vi "Analog Gen Cfg Popup.vi"(8 "error in (no error)":errorcluster, 11 "config file in":path caption="Configuration File") -> (0 "error out":errorcluster, 3 "config file out":path caption="Configuration File")   [LabVIEW 2021, in "Audio Popup UI.lvlib"]
uses:
  Audio Popup UI.lvlib
  service/generation/controls/analog output settings.ctl
  service/generation/controls/terminal configuration.ctl
  <vilib>/Utility/miscctls.llb/LVPointTypeDef.ctl
  analog gen settings/Analog Gen Settings.lvlib
  service/generation/controls/AudioGenTypeDefs.lvlib
panel:
  in  "terminal configuration":T1 caption="Terminal configuration"
  in  "range":dbl=2.0 caption="Output range"
  out "output settings":T2={"output rate"=0.0, "range"=0.0, "terminal configuration"=enum."Pseudodifferential", "output impedance"=0.0, "common mode offset"=0.0, "pure tone mode"=FALSE}
  in  "Save":bool
  in  "output rate":dbl=2.0 caption="Output rate"
  # "Analog Output Configuration"
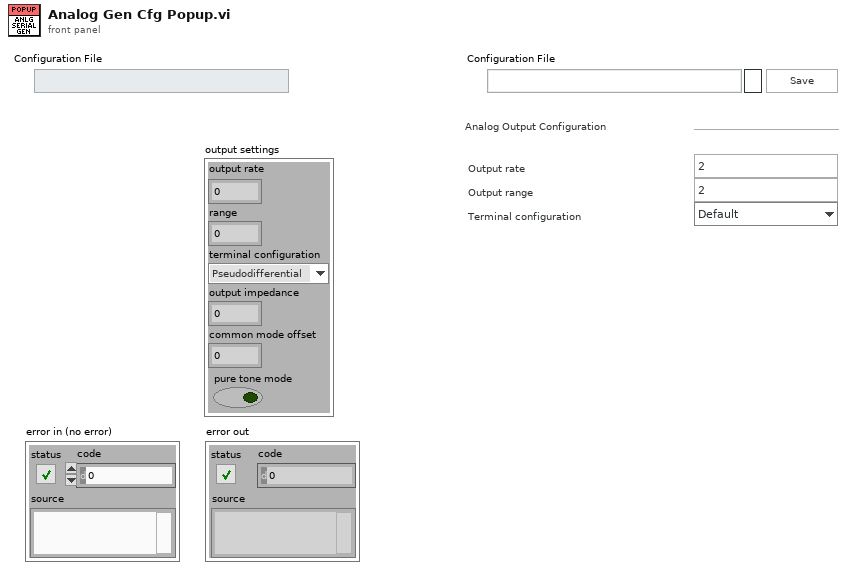
[diagram p1: front panel]
types:
  T1 = typedef "AudioGenTypeDefs.lvlib/terminal configuration.ctl" = enum32{"Default", "RSE", "Differential", "Pseudodifferential"}
  T2 = typedef "AudioGenTypeDefs.lvlib/analog output settings.ctl" = cluster{"output rate":dbl, "range":dbl, "terminal configuration":T1, "output impedance":dbl, "common mode offset":dbl, "pure tone mode":bool}
  T3 = typedef "LVPointTypeDef.ctl" = cluster{"Horizontal":i16, "Vertical":i16}
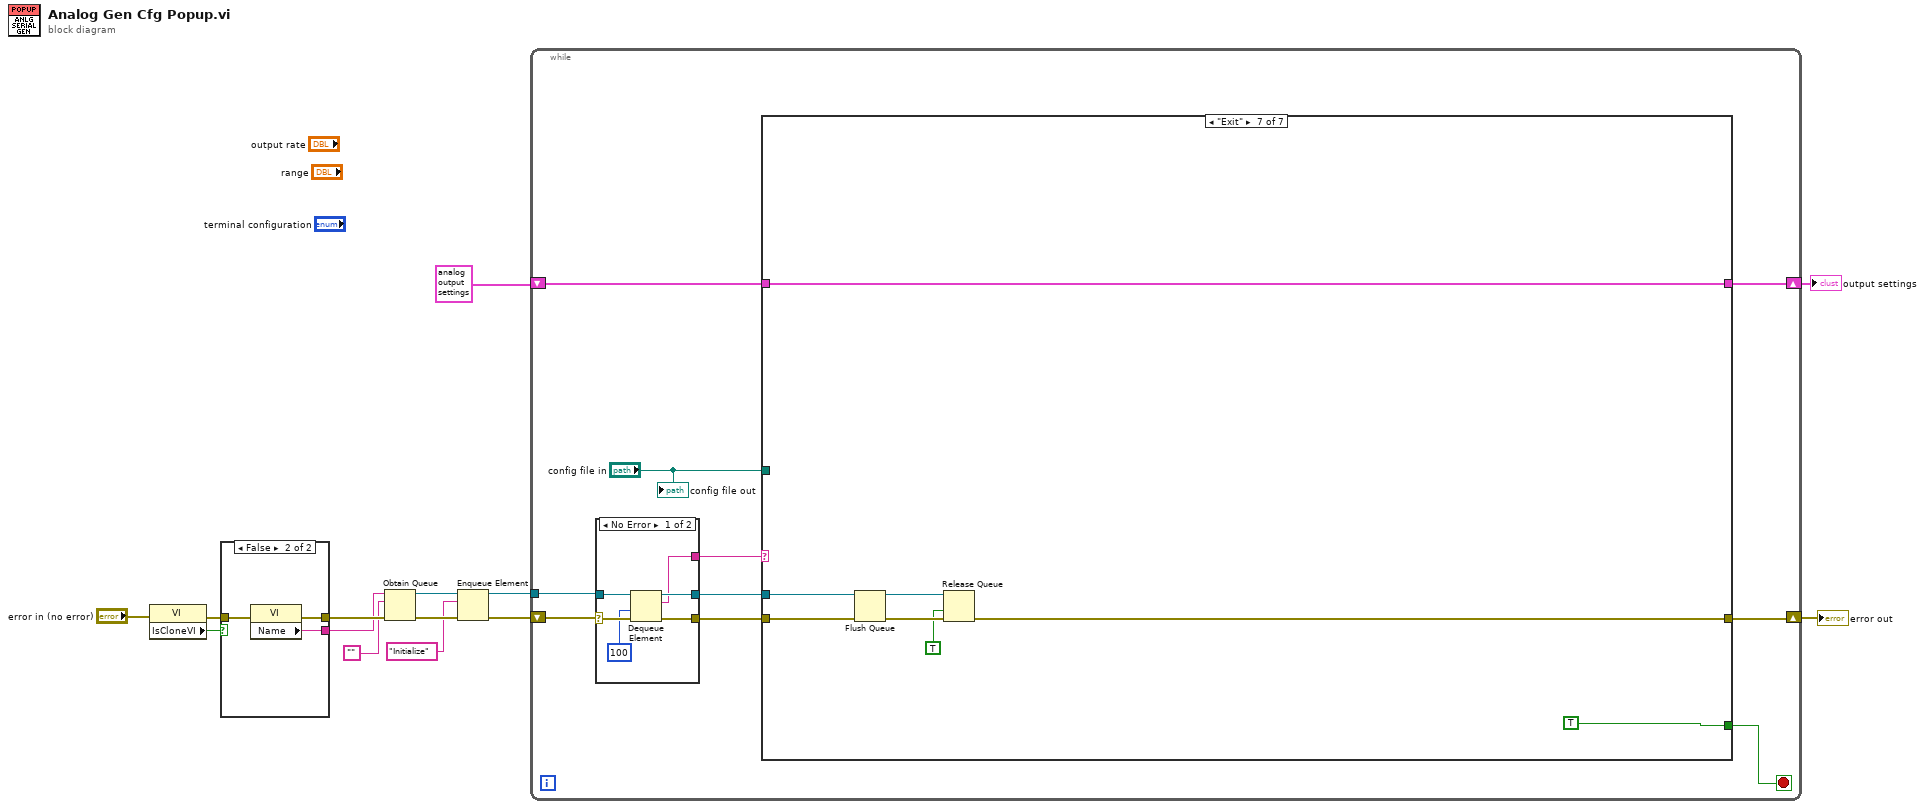
[diagram p0: block diagram]
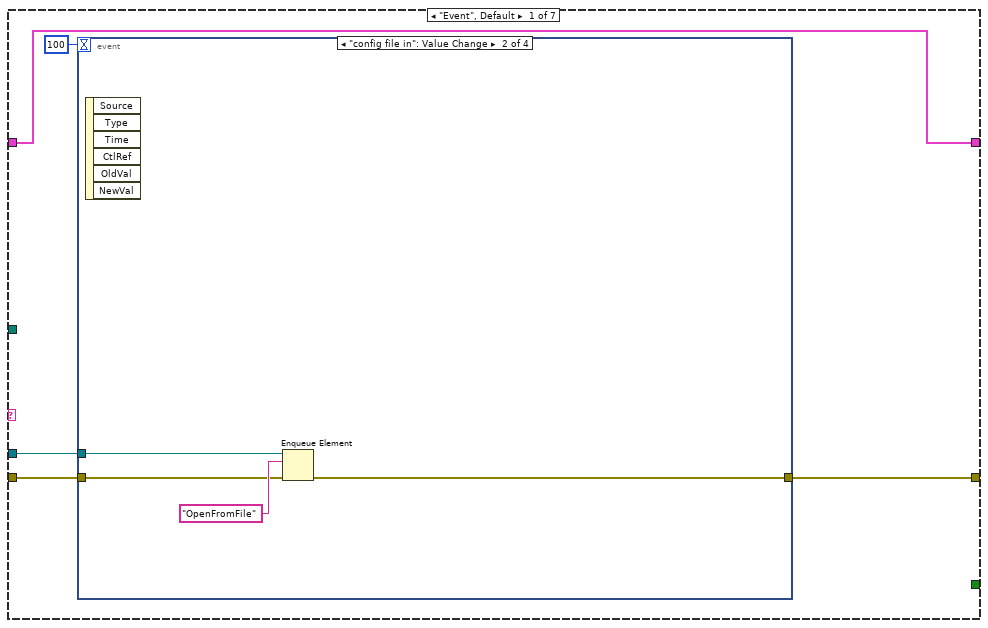
[diagram p2: hidden frame]
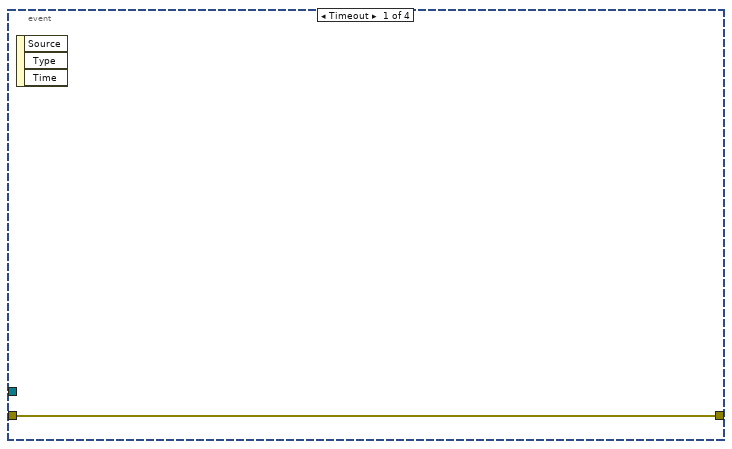
[diagram p3: hidden frame]
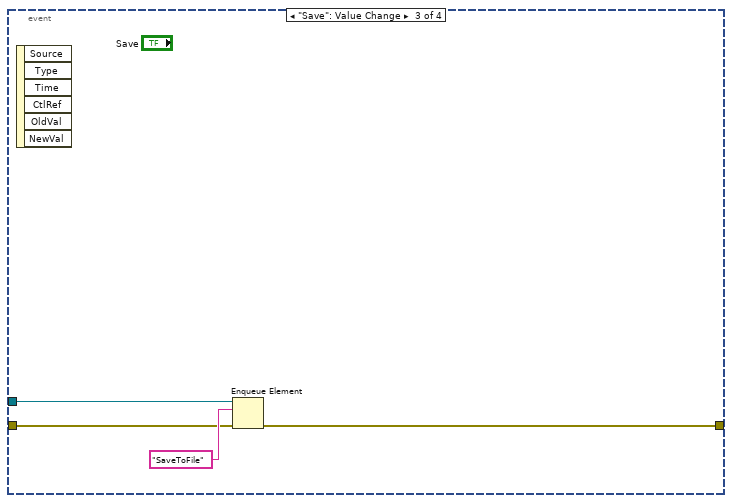
[diagram p4: hidden frame]
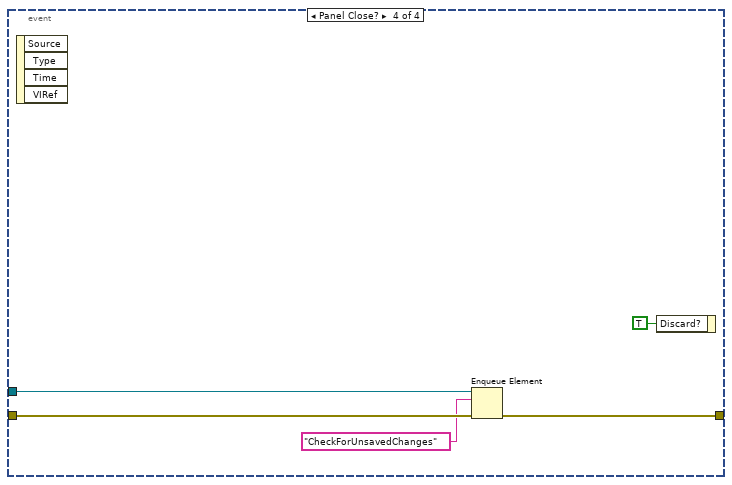
[diagram p5: hidden frame]
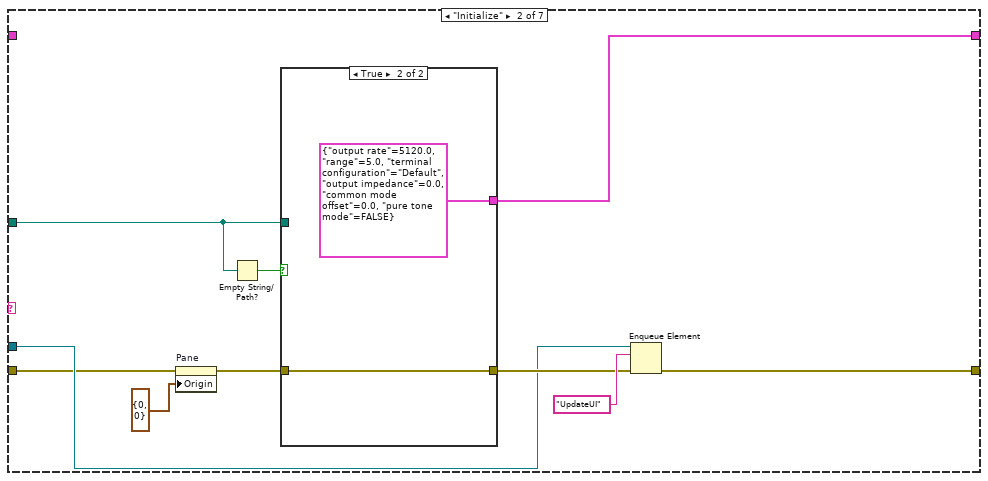
[diagram p6: hidden frame]
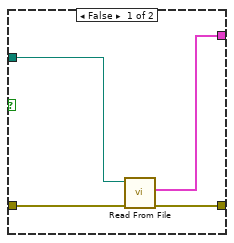
[diagram p7: hidden frame]
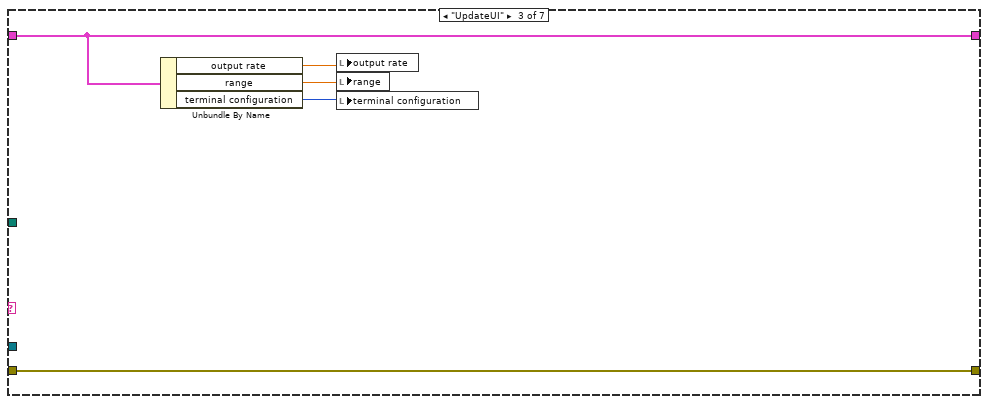
[diagram p8: hidden frame]
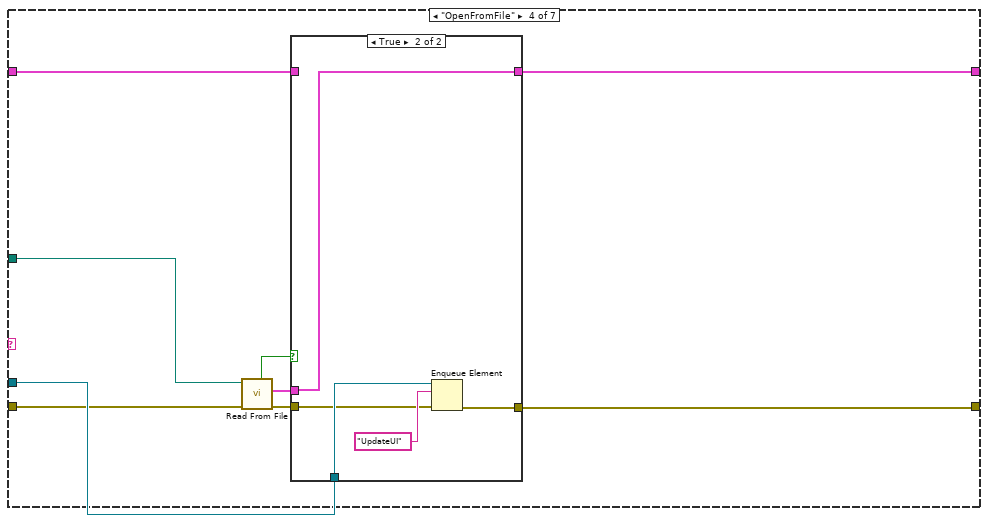
[diagram p9: hidden frame]
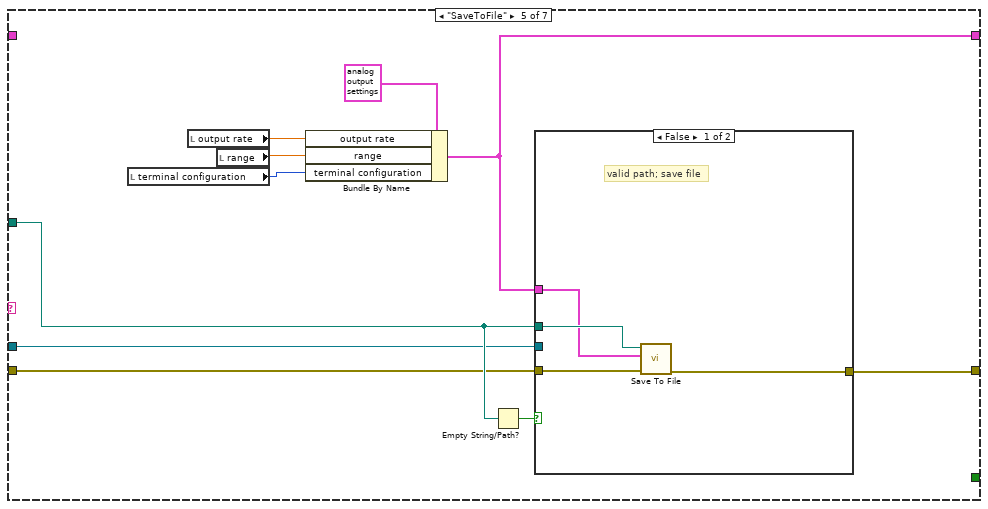
[diagram p11: hidden frame]
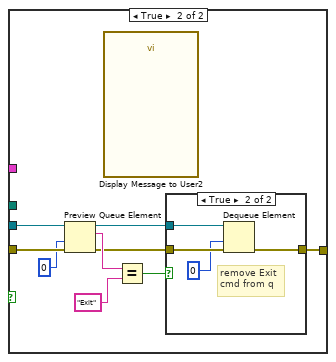
[diagram p12: hidden frame]
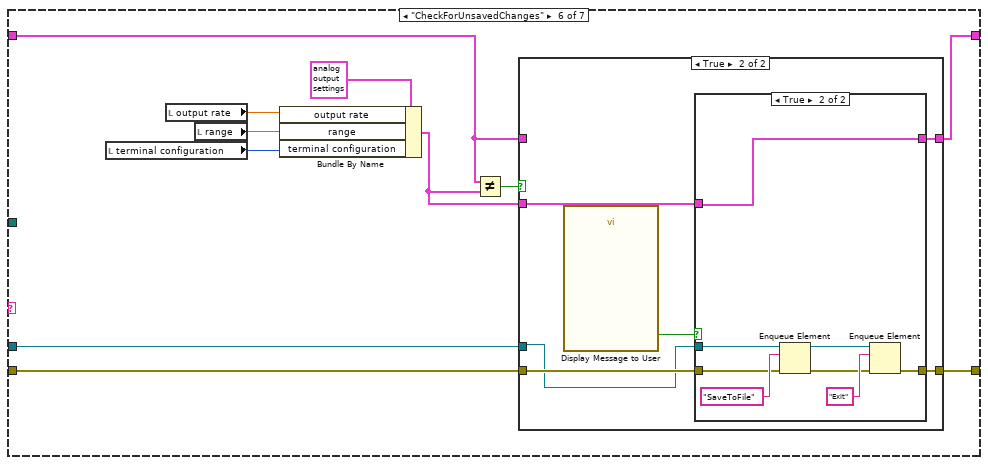
[diagram p14: hidden frame]
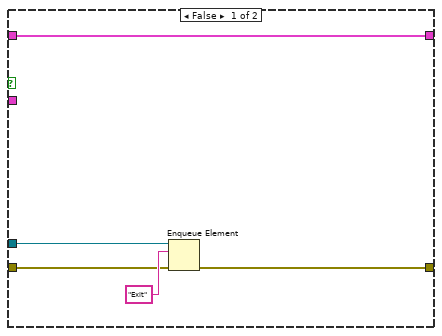
[diagram p15: hidden frame]
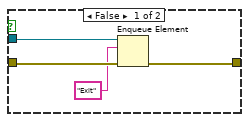
[diagram p16: hidden frame]
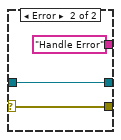
[diagram p17: hidden frame]
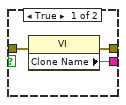
[diagram p18: hidden frame]
diagram:
  n1 = property class="VI"(error in="error in (no error)") -> (error out=w7:errorcluster, "IsCloneVI"=w8:bool)  [unwired: 1 in, 1 out]
  n2 = case shown="False" w8 {
    tunnel: [w17 w20] -> w14
    tunnel: [w16 w19] -> w13
    tunnel: w7 -> [w15 w18]
    frame True {
      n3 = property class="VI"(error in=w15) -> (error out=w17:errorcluster, "Clone Name"=w16:string)  [unwired: 1 in, 1 out]
    }
    frame False {
      n4 = property class="VI"(error in=w18) -> (error out=w20:errorcluster, "Name"=w19:string)  [unwired: 1 in, 1 out]
    }
  }
  n5 = Obtain Queue(name (unnamed)=w13, element data type="", error in (no error)=w14) -> (queue out=w11:refnum<queue>, error out=w12:errorcluster)  [unwired: 2 in, 1 out]
  n6 = Enqueue Element(queue=w11, element="Initialize", error in (no error)=w12) -> (queue out=w5:refnum<queue>, error out=w6:errorcluster)  [unwired: 1 in, 1 out]
  n7 = while {
    tunnel: w5 -> [w29]
    shift-right: [w25] -> w4
    shift-left: w6 -> [w30]
    shift-right: [w22] -> w1
    shift-left: T2 {"output rate"=51200.0, "range"=5.0, "terminal configuration"=enum."Pseudodifferential", "output impedance"=0.0, "common mode offset"=0.0, "pure tone mode"=FALSE} ("output settings") -> [w23]
    stop <- w24 stop-if-true
    n8 = case shown="No Error" w30 {
      selector: w30 -> [w162 w165]
      tunnel: [w161 w165] -> w26
      tunnel: w29 -> [w160 w164]
      tunnel: [w159 w164] -> w27
      tunnel: [w158 "Handle Error"] -> w28
      frame No Error {
        n9 = Dequeue Element(queue=w160, timeout in ms (-1)=100, error in (no error)=w162) -> (queue out=w159:refnum<queue>, element=w158:string, error out=w161:errorcluster)  [unwired: 1 out]
      }
      frame Error {
      }
    }
    n10 = case shown="\"Exit\"" w28 {
      tunnel: w27 -> [w33 w53 _ w79 w91 w121 w152]
      tunnel: w26 -> [w34 w51 w70 w76 w93 w124 w153]
      tunnel: [w32 w54 w70 w78 w96 w123 w150] -> w25
      tunnel: [_ _ _ _ _ _ TRUE] -> w24
      tunnel: w23 -> [w31 _ w69 w73 _ w119 w149]
      tunnel: [w31 w57 w69 w72 w95 w122 w149] -> w22
      tunnel: "config file in" -> [_ w58 _ w77 w94 _ _]
      frame "Event", Default {
        n11 = event shown="[1] \"config file in\": Value Change" {
          selector: _ -> [_ _ _ _]
          dyn-events: _ -> [_ _ _ _]
          timeout: 100 -> [_ _ _ _]
          tunnel: w34 -> [w36 w39 w43 w48]
          tunnel: w33 -> [_ w38 w42 w47]
          tunnel: [w36 w37 w41 w46] -> w32
          event Timeout {
            n12 = event-data() -> ()  [unwired: 1 in, 3 out]
          }
          event "config file in": Value Change {
            n13 = event-data() -> ()  [unwired: 1 in, 6 out]
            n14 = Enqueue Element(queue=w38, element="OpenFromFile", error in (no error)=w39) -> (error out=w37:errorcluster)  [unwired: 1 in, 2 out]
          }
          event "Save": Value Change {
            n15 = event-data() -> ()  [unwired: 1 in, 6 out]
            n16 = Enqueue Element(queue=w42, element="SaveToFile", error in (no error)=w43) -> (error out=w41:errorcluster)  [unwired: 1 in, 2 out]
          }
          event Panel Close? {
            n17 = event-data() -> ()  [unwired: 1 in, 4 out]
            n18 = Enqueue Element(queue=w47, element="CheckForUnsavedChanges", error in (no error)=w48) -> (error out=w46:errorcluster)  [unwired: 1 in, 2 out]
            n19 = event-data("Discard?"=TRUE) -> ()  [unwired: 1 in, 1 out]
          }
        }
      }
      frame "Initialize" {
        n20 = property on="Pane" class="Pane"(error in=w51, "Origin"=T3 {"Horizontal"=0, "Vertical"=0}) -> (error out=w50:errorcluster)  [unwired: 1 in, 1 out]
        n21 = Empty String/Path?(string/path=w58) -> (empty?=w59:bool)
        n22 = case shown="True" w59 {
          tunnel: w50 -> [w63 w65]
          tunnel: w58 -> [w62 _]
          tunnel: [w60 T2 {"output rate"=5120.0, "range"=5.0, "terminal configuration"=enum."Default", "output impedance"=0.0, "common mode offset"=0.0, "pure tone mode"=FALSE} ("analog generation")] -> w57
          tunnel: [w61 w65] -> w55
          frame False {
            n23 = call "Read From File.vi"("error in (no error)"=w63, "file path"=w62) -> ("error out"=w61:errorcluster, "analog generation"=w60:T2)  [unwired: 7 in, 1 out]
          }
          frame True {
          }
        }
        n24 = Enqueue Element(queue=w53, element="UpdateUI", error in (no error)=w55) -> (error out=w54:errorcluster)  [unwired: 1 in, 2 out]
      }
      frame "UpdateUI" {
        n25 = Unbundle By Name(w69) -> ("output rate"=w68:dbl, "range"=w67:dbl, "terminal configuration"=w66:T1)
        n26 = local write "output rate"(w68) -> ()
        n27 = local write "range"(w67) -> ()
        n28 = local write "terminal configuration"(w66) -> ()
      }
      frame "OpenFromFile" {
        n29 = call "Read From File.vi"("error in (no error)"=w76, "file path"=w77) -> ("error out"=w75:errorcluster, "analog generation"=w71:T2, "file exists?"=w74:bool)  [unwired: 7 in]
        n30 = case shown="True" w74 {
          tunnel: w79 -> [_ w85]
          tunnel: [w80 w84] -> w78
          tunnel: w75 -> [w80 w83]
          tunnel: w73 -> [w81 _]
          tunnel: [w81 w82] -> w72
          tunnel: w71 -> [_ w82]
          frame False {
          }
          frame True {
            n31 = Enqueue Element(queue=w85, element="UpdateUI", error in (no error)=w83) -> (error out=w84:errorcluster)  [unwired: 1 in, 2 out]
          }
        }
      }
      frame "SaveToFile" {
        n32 = local read "terminal configuration"() -> (w87:T1)
        n33 = local read "output rate"() -> (w89:dbl)
        n34 = local read "range"() -> (w88:dbl)
        n35 = Bundle By Name(cluster=T2 {"output rate"=51200.0, "range"=5.0, "terminal configuration"=enum."Pseudodifferential", "output impedance"=0.0, "common mode offset"=0.0, "pure tone mode"=FALSE} ("output settings"), "output rate"=w89, "range"=w88, "terminal configuration"=w87) -> (w95:T2)
        n36 = Empty String/Path?(string/path=w94) -> (empty?=w92:bool)
        n37 = case shown="False" w92 {
          tunnel: [w100 w102] -> w96
          tunnel: w95 -> [w97 _]
          tunnel: w94 -> [w99 _]
          tunnel: w93 -> [w98 w109]
          tunnel: w91 -> [_ w108]
          frame False {
            # "valid path; save file"
            n38 = call "Save To File.vi"("error in (no error)"=w98, "output settings"=w97, "file path"=w99) -> ("error out"=w100:errorcluster)  [unwired: 8 in]
          }
          frame True {
            n39 = Preview Queue Element(queue=w108, timeout in ms (-1)=0, error in (no error)=w109) -> (queue out=w105:refnum<queue>, element=w107:string, error out=w103:errorcluster)  [unwired: 1 out]
            n40 = call "Display Message to User2"() -> ()  [unwired: 10 in, 2 out]
            n41 = Equal?(x=w107, y="Exit") -> (x = y?=w104:bool)
            n42 = case shown="True" w104 {
              tunnel: w105 -> [_ w114]
              tunnel: w103 -> [w110 w113]
              tunnel: [w110 w112] -> w102
              frame False {
              }
              frame True {
                # "remove Exit\ncmd from q"
                n43 = Dequeue Element(queue=w114, timeout in ms (-1)=0, error in (no error)=w113) -> (error out=w112:errorcluster)  [unwired: 3 out]
              }
            }
          }
        }
      }
      frame "CheckForUnsavedChanges" {
        n44 = local read "terminal configuration"() -> (w117:T1)
        n45 = local read "output rate"() -> (w115:dbl)
        n46 = local read "range"() -> (w116:dbl)
        n47 = Bundle By Name(cluster=T2 {"output rate"=51200.0, "range"=5.0, "terminal configuration"=enum."Pseudodifferential", "output impedance"=0.0, "common mode offset"=0.0, "pure tone mode"=FALSE} ("output settings"), "output rate"=w115, "range"=w116, "terminal configuration"=w117) -> (w120:T2)
        n48 = Not Equal?(x=w119, y=w120) -> (x != y?=w125:bool)
        n49 = case shown="True" w125 {
          tunnel: w124 -> [w128 w136]
          tunnel: [w126 w132] -> w123
          tunnel: w120 -> [_ w134]
          tunnel: w119 -> [w130 _]
          tunnel: [w130 w133] -> w122
          tunnel: w121 -> [w127 w131]
          frame False {
            n50 = Enqueue Element(queue=w127, element="Exit", error in (no error)=w128) -> (error out=w126:errorcluster)  [unwired: 1 in, 2 out]
          }
          frame True {
            n51 = call "Display Message to User"() -> ("Yes"=w135:bool)  [unwired: 10 in, 1 out]
            n52 = case shown="True" w135 {
              tunnel: w136 -> [w140 w147]
              tunnel: w134 -> [_ w146]
              tunnel: [_ w146] -> w133
              tunnel: [w138 w142] -> w132
              tunnel: w131 -> [w139 w141]
              frame False {
                n53 = Enqueue Element(queue=w139, element="Exit", error in (no error)=w140) -> (error out=w138:errorcluster)  [unwired: 1 in, 2 out]
              }
              frame True {
                n54 = Enqueue Element(queue=w141, element="SaveToFile", error in (no error)=w147) -> (queue out=w143:refnum<queue>, error out=w144:errorcluster)  [unwired: 1 in, 1 out]
                n55 = Enqueue Element(queue=w143, element="Exit", error in (no error)=w144) -> (error out=w142:errorcluster)  [unwired: 1 in, 2 out]
              }
            }
          }
        }
      }
      frame "Exit" {
        n56 = Flush Queue(queue=w152, error in (no error)=w153) -> (queue out=w156:refnum<queue>, error out=w155:errorcluster)  [unwired: 1 out]
        n57 = Release Queue(queue=w156, force destroy? (F)=TRUE, error in (no error)=w155) -> (error out=w150:errorcluster)  [unwired: 2 out]
      }
    }
    "config file out" <- "config file in"
  }
  "error out" <- w4
  "output settings" <- w1
